vi "append_table.vi"() -> ()   [LabVIEW 2014]
uses:
  <vilib>/Utility/NIReport.llb/Append Text Table to Report (wrap).vi
  <vilib>/Utility/NIReport.llb/NI_report.lvclass
panel:
  in  "text data":string[][](array[string])
  in  "row headers":string[](array[string])
  in  "column headers":string[](array[string])
  in  "template (empty)":path
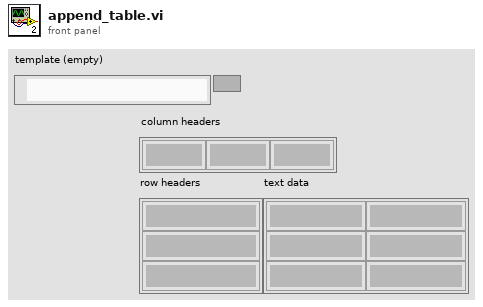
[diagram p1: front panel]
types:
  T1 = enum16{"Standard Report", "HTML", "Word", "Excel"}
  T2 = enum16{"maximized", "minimized", "normal", "no change"}
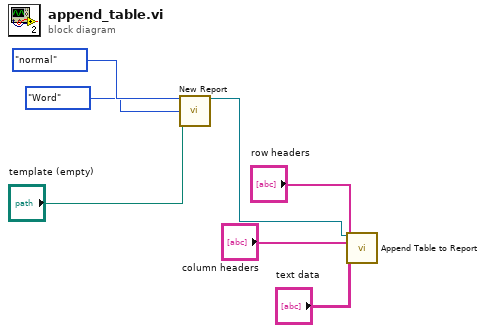
[diagram p0: block diagram]
diagram:
  n1 = call <vilib>:"New Report.vi"("window state (normal)"=T2."normal", "report type"=T1."Word", "template (empty)"="template (empty)") -> ("report out"=w4:refnum<class "NI_report.lvclass">)  [unwired: 11 in, 1 out]
  n2 = call-poly <vilib>:"Append Table to Report.vi"("report in"=w4, "column headers"="column headers", "row headers"="row headers", "text data"="text data") -> ()  [unwired: 8 in, 4 out]
